vi "Create and Add Tasks.vi"(8 "error in (no error)":errorcluster, 11 "HAL GOOP4:Series Base in":refnum<class "Series Base.lvclass">) -> (0 "error out":errorcluster, 3 "HAL GOOP4:Series Base out":refnum<class "Series Base.lvclass">)   [LabVIEW 2023, in "HAL GOOP4.lvlib" / "Series Base.lvclass"]
uses:
  Series Base.lvclass
  Series Base.lvclass/Series Base.ctl
  Task/Task Base/Task Base.lvclass
  Task/Task Base/Task Base.lvclass/Task Base.ctl
  <vilib>/Utility/miscctls.llb/LVMapReplaceAction.ctl
  b874e428-42f4-4ebe-8b0a-882075bdcbe6.vi
  <vilib>/JDP Science/JSONtext/Find Item.vi
  <vilib>/JDP Science/JSONtext/Next JSON Value.vi
  <vilib>/JDP Science/JSONtext/String Subset.vi
  <vilib>/JDP Science/JSONtext/Parsing/Advance past next JSON Value (inlined COPY).vi
  <vilib>/JDP Science/JSONtext/Parsing/Advance past whitespace.vi
  <vilib>/JDP Science/JSONtext/Parsing/Advance past String.vi
  <vilib>/JDP Science/JSONtext/Parsing/Advance past Number.vi
  <vilib>/JDP Science/JSONtext/Parsing/Advance past Line Ending.vi
  <vilib>/JDP Science/JSONtext/Parsing/Parse Full Path or Item Name.vi
  <vilib>/JDP Science/JSONtext/Parsing/Advance past Array.vi
  <vilib>/JDP Science/JSONtext/Parsing/Advance past Object.vi
  <vilib>/JDP Science/JSONtext/support/Error Cluster From Code.vi
  <vilib>/JDP Science/JSONtext/Offset/Find Item Locations by Path.vi
  <vilib>/JDP Science/JSONtext/JSON text to Variant.vi
  <vilib>/Utility/error.llb/Error Cluster From Error Code.vi
  <vilib>/JDP Science/JSONtext/LVClass Serializer/JSONtext LVClass Serializer.lvclass
  <vilib>/ErrorRing/Error Ring.xnode
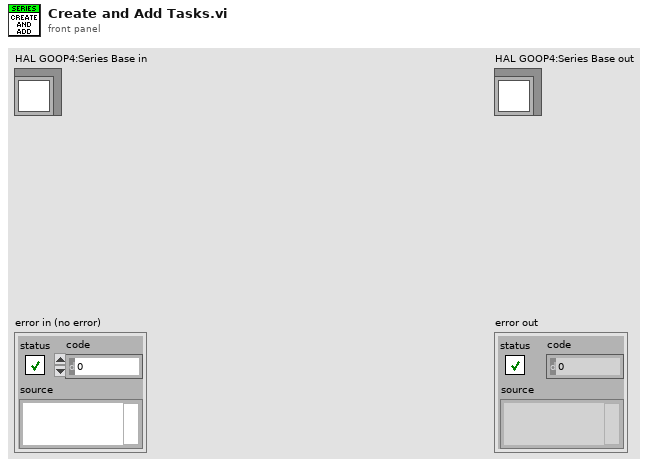
[diagram p1: front panel]
types:
  T1 = typedef "LVMapReplaceAction.ctl" = enum32{"Modify Entry only if found", "Add or Modify Entry", "Delete Entry"}
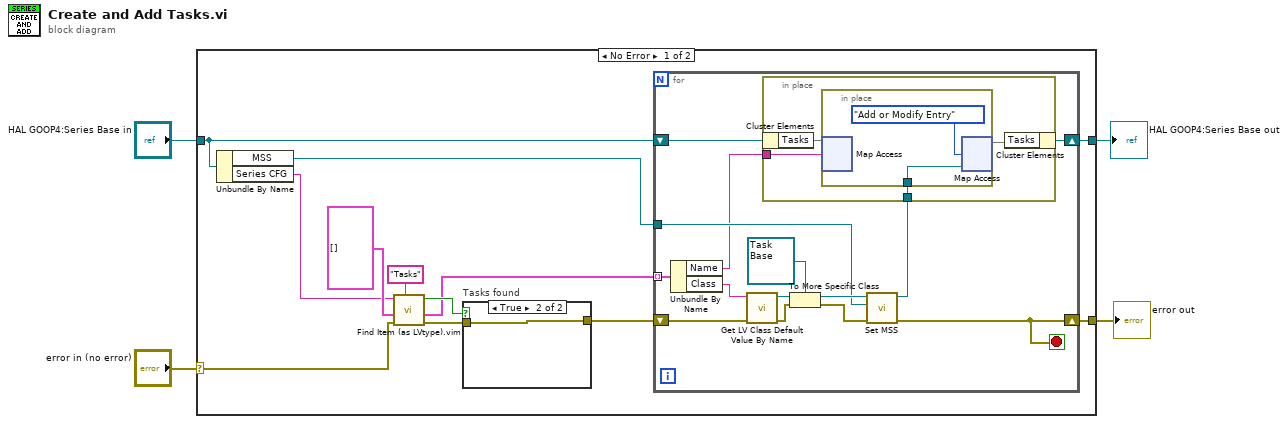
[diagram p0: block diagram]
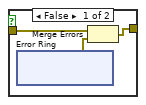
[diagram p2: hidden frame]
diagram:
  n1 = case shown="No Error" "error in (no error)" {
    selector: "error in (no error)" -> [w15 w47]
    tunnel: [w9 w47] -> w3
    tunnel: [w8 w46] -> w1
    tunnel: "HAL GOOP4:Series Base in" -> [w7 w46]
    frame No Error {
      n2 = Unbundle By Name(w7) -> ("MSS"=w6:refnum<class "Measure and Stimulus Subsystems.lvclass">, "Series CFG"=w5:string)
      n3 = call "Find Item (as LVtype).vim"("$Path or Item Name"="Tasks", "error in (no error)"=w15, "Data Type and Default Value"=cluster{"Name":string, "Class":string}[] [] ("Tasks"), "JSON"=w5) -> ("error out"=w12:errorcluster, "Data"=w11:cluster{"Name":string, "Class":string}[], "Found"=w13:bool)  [unwired: 4 in, 1 out]
      n4 = case "Tasks found" shown="True" w13 {
        tunnel: w12 -> [w39 w45]
        tunnel: [w38 w45] -> w10
        frame False {
          n5 = xnode "Error Ring"() -> ("error out"=w37:errorcluster)
          n6 = Merge Errors(w39, w37) -> (w38:errorcluster)
        }
        frame True {
        }
      }
      n7 = for {
        tunnel: w11 -> [w27] mode=indexing
        shift-right: [w17] -> w9
        shift-left: w10 -> [w26]
        tunnel: w6 -> [w21]
        shift-right: [w18] -> w8
        shift-left: w7 -> [w24]
        stop <- w17 stop-if-true
        n8 = Unbundle By Name(w27) -> ("Name"=w19:string, "Class"=w25:string)
        n9 = call <vilib>:"Get LV Class Default Value By Name.vi"("error in (no error)"=w26, "class name"=w25) -> ("error out"=w30:errorcluster, "object"=w29:refnum<class>)  [unwired: 8 in]
        n10 = To More Specific Class(target class=refnum<class "Task Base.lvclass"> refnum ("HAL GOOP4.lvlib:Task Base.lvclass"), reference=w29, error in=w30) -> (specific class reference=w23:refnum<class "Task Base.lvclass">, error out=w22:errorcluster)
        n11 = call "Set MSS.vi"("error in (no error)"=w22, "MSS"=w21, "Task Base in"=w23) -> ("error out"=w17:errorcluster, "Task Base out"=w20:refnum<class "Task Base.lvclass">)  [unwired: 7 in]
        n12 = in-place {
          in-place-border: w20 -> [w33]
          in-place-border: w19 -> [w32]
          n13 = in-place-cluster #1(w24) -> ("Tasks"=w34:map{string, refnum<class "Task Base.lvclass">})
          n14 = in-place {
            in-place-border: w33 -> [w36]
            n15 = in-place-map #2(w34, w32) -> ()  [unwired: 1 in, 2 out]
            n16 = in-place-map #2(w36, LVMapReplaceAction."Add or Modify Entry" ("action")) -> (w31:map{string, refnum<class "Task Base.lvclass">})  [unwired: 2 out]
          }
          n17 = in-place-cluster #1("Tasks"=w31) -> (w18:refnum<class "Series Base.lvclass">)
        }
      }
    }
    frame Error {
    }
  }
  "error out" <- w3
  "HAL GOOP4:Series Base out" <- w1
